vi "DAC Run.vi"(8 "error in":errorcluster, 11 "DAC Pressure Scan in":refnum<class "DAC Pressure Scan.lvclass">) -> (0 "error out":errorcluster, 3 "DAC Pressure Scan out":refnum<class "DAC Pressure Scan.lvclass">)   [LabVIEW 2019, in "DAC.lvlib" / "DAC Pressure Scan.lvclass"]
uses:
  DAC Pressure Scan.lvclass
  C:/Users/wg/Documents/LV_Projects/test-stand/App/DAC/DAC.lvclass
  DAC.lvclass/DAC.ctl
  Results/Results Method.ctl
  Results/Water Tunnel Results/Water Tunnel Results.lvclass
  DAC Pressure Scan.lvclass/DAC Pressure Scan.ctl
  <vilib>/DAQmx/read.llb/DAQmx Read (Analog 1D Wfm NChan 1Samp).vi
  <vilib>/DAQmx/miscellaneous.llb/DAQmx Fill In Error Info.vi
  DAC.lvclass
  Results/Results.lvlib
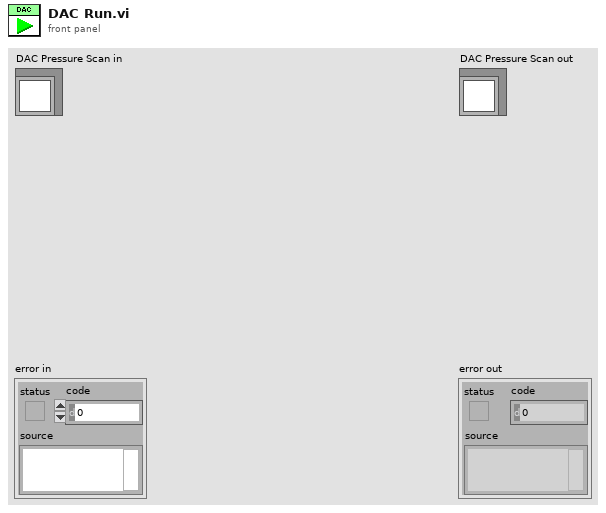
[diagram p1: front panel]
types:
  T1 = typedef "Results.lvlib/Results Method.ctl" = enum16{"Get", "Set"}
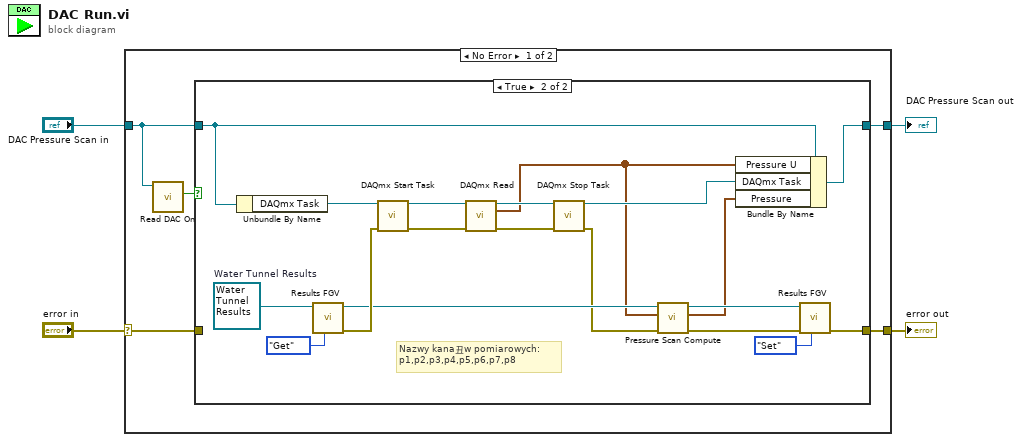
[diagram p0: block diagram]
diagram:
  n1 = case shown="No Error" "error in" {
    selector: "error in" -> [w7 w32]
    tunnel: [w6 w32] -> w2
    tunnel: [w8 w31] -> w1
    tunnel: "DAC Pressure Scan in" -> [w5 w31]
    frame No Error {
      n2 = call "Read DAC On.vi"("DAC in"=w5) -> ("DAC On"=w9:bool)  [unwired: 8 in, 2 out]
      n3 = case shown="True" w9 {
        tunnel: w5 -> [w11 w25]
        tunnel: [w11 w21] -> w8
        tunnel: w7 -> [w10 _]
        tunnel: [w10 w20] -> w6
        frame False {
        }
        frame True {
          w18 = refnum<class "Water Tunnel Results.lvclass"> refnum  # Water Tunnel Results
          # "Nazwy kana丑w pomiarowych:\np1,p2,p3,p4,p5,p6,p7,p8"
          n4 = Unbundle By Name(w25) -> ("DAQmx Task"=w30:refnum<k21>)
          n5 = call-dynamic "Results FGV.vi"("Method"=Results_Method."Get", "Water Tunnel Results in"=w18) -> ("error out"=w22:errorcluster, "Water Tunnel  Results out"=w17:refnum<class "Water Tunnel Results.lvclass">)  [unwired: 8 in]
          n6 = call <vilib>:"DAQmx Start Task.vi"("task/channels in"=w30, "error in"=w22) -> ("task out"=w29:refnum<k21>, "error out"=w27:errorcluster)  [unwired: 12 in]
          n7 = call-poly <vilib>:"DAQmx Read.vi"("task/channels in"=w29, "error in"=w27) -> ("task out"=w28:refnum<k21>, "data"=w12:waveform(dbl)[], "error out"=w26:errorcluster)  [unwired: 11 in]
          n8 = call <vilib>:"DAQmx Stop Task.vi"("task/channels in"=w28, "error in"=w26) -> ("task out"=w19:refnum<k21>, "error out"=w16:errorcluster)  [unwired: 12 in]
          n9 = call "Pressure Scan Compute.vi"("error in"=w16, "Pressure U"=w12, "Water Tunnel Results in"=w17) -> ("error out"=w14:errorcluster, "Pressure"=w13:waveform(dbl)[], "Water Tunnel Results out"=w15:refnum<class "Water Tunnel Results.lvclass">)  [unwired: 6 in]
          n10 = Bundle By Name(cluster=w25, "Pressure U"=w12, "DAQmx Task"=w19, "Pressure"=w13) -> (w21:refnum<class "DAC Pressure Scan.lvclass">)
          n11 = call-dynamic "Results FGV.vi"("Method"=Results_Method."Set", "error in"=w14, "Water Tunnel Results in"=w15) -> ("error out"=w20:errorcluster)  [unwired: 7 in, 1 out]
        }
      }
    }
    frame Error {
    }
  }
  "error out" <- w2
  "DAC Pressure Scan out" <- w1
